vi "subGetDependenciesForProjectItems.vi"(7 "Shallow check":bool, 8 "error in (no error)":errorcluster, 9 "Dependents":refnum<vi>[](array[refnum]), 10 "Owning project":path, 11 "SolutionBuilder in":refnum<class "SolutionBuilder.lvclass">) -> (0 "error out":errorcluster, 3 "SolutionBuilder out":refnum<class "SolutionBuilder.lvclass">)   [LabVIEW 2020, in "SolutionBuilder.lvlib" / "SolutionBuilder.lvclass"]
uses:
  SolutionBuilder.lvclass
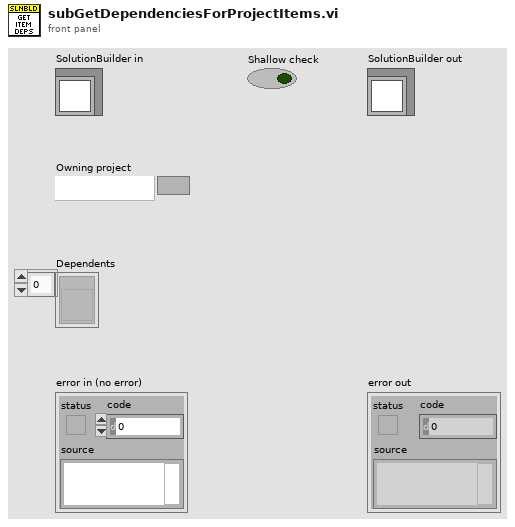
[diagram p1: front panel]
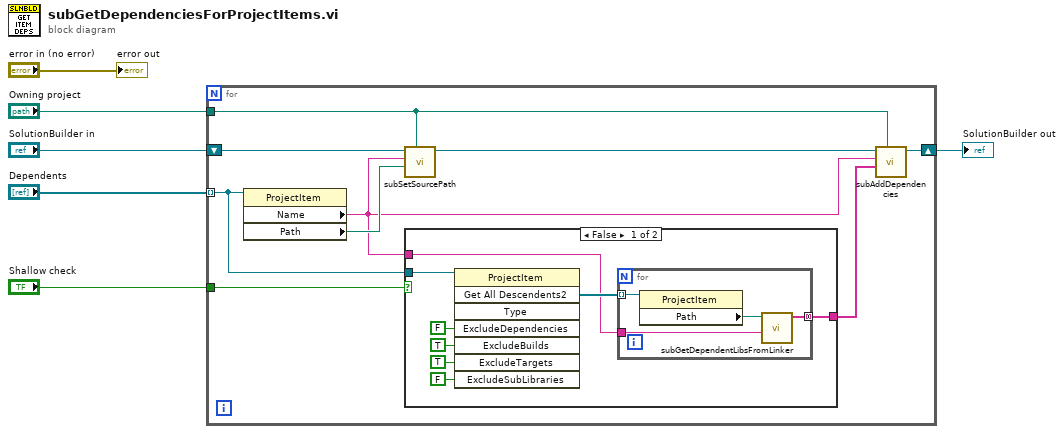
[diagram p0: block diagram]
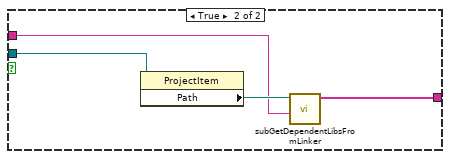
[diagram p2: hidden frame]
diagram:
  n1 = for {
    tunnel: "Dependents" -> [w9] mode=indexing
    shift-right: [w12] -> w4
    shift-left: "SolutionBuilder in" -> [w15]
    tunnel: "Owning project" -> [w11]
    tunnel: "Shallow check" -> [w7]
    n2 = property class="ProjectItem"(reference=w9) -> ("Name"=w8:string, "Path"=w14:path)  [unwired: 1 in, 2 out]
    n3 = call "subSetSourcePath.vi"("Project path"=w11, "ProjectItem path"=w14, "Name"=w8, "SolutionBuilder in"=w15) -> ("SolutionBuilder out"=w13:refnum<class "SolutionBuilder.lvclass">)  [unwired: 6 in, 1 out]
    n4 = case shown="False" w7 {
      tunnel: [w18 w29] -> w10
      tunnel: w9 -> [w17 w30]
      tunnel: w8 -> [w16 w28]
      frame False {
        n5 = invoke class="ProjectItem" method="Get All Descendents2"(reference=w17, "ExcludeDependencies"=FALSE, "ExcludeBuilds"=TRUE, "ExcludeTargets"=TRUE, "ExcludeSubLibraries"=FALSE) -> ("Get All Descendents2"=w19:refnum<vi>[])  [unwired: 3 in, 7 out]
        n6 = for {
          tunnel: w19 -> [w27] mode=indexing
          tunnel: [w26] -> w18 mode=concatenating
          tunnel: w16 -> [w24]
          n7 = property class="ProjectItem"(reference=w27) -> ("Path"=w25:path)  [unwired: 1 in, 2 out]
          n8 = call "subGetDependentLibsFromLinker.vi"("Name"=w24, "Path"=w25) -> ("Dependent libs"=w26:string[])  [unwired: 8 in, 1 out]
        }
      }
      frame True {
        n9 = property class="ProjectItem"(reference=w30) -> ("Path"=w31:path)  [unwired: 1 in, 2 out]
        n10 = call "subGetDependentLibsFromLinker.vi"("Name"=w28, "Path"=w31) -> ("Dependent libs"=w29:string[])  [unwired: 8 in, 1 out]
      }
    }
    n11 = call "subAddDependencies.vi"("Project path"=w11, "Dependencies"=w10, "Name"=w8, "SolutionBuilder in"=w13) -> ("SolutionBuilder out"=w12:refnum<class "SolutionBuilder.lvclass">)  [unwired: 6 in, 1 out]
  }
  "SolutionBuilder out" <- w4
  "error out" <- "error in (no error)"
